vi "Step.vi"(8 "error in (no error)":errorcluster, 11 "SQL Statement in":refnum<class "SQL Statement.lvclass">) -> (0 "error out":errorcluster, 2 "Row returned":bool, 3 "SQL Statement out":refnum<class "SQL Statement.lvclass">)   [LabVIEW 2023, in "SQLiteSupport.lvlib" / "SQL Statement.lvclass"]
doc: "Steps to another row of a multiple-row returned data set. Please use \"First Step\" to actually execute the statement (and return the first row), rather than \"Step\"."
uses:
  SQL Statement.lvclass
panel:
  # "Step, and anything containing Step, may block while\nwaiting for another operation to unlock the database,\nand thus must be reentrant in order to prevent lock-up."
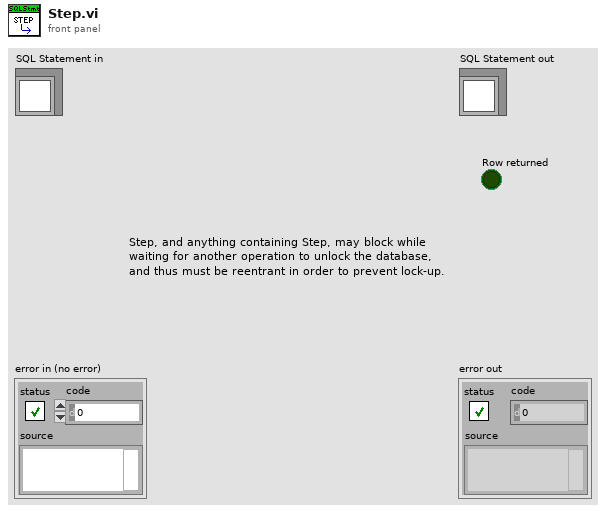
[diagram p1: front panel]
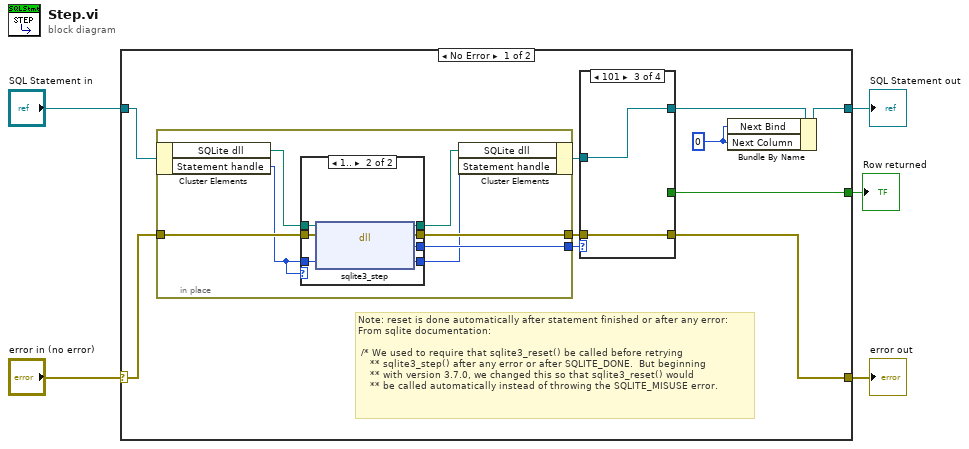
[diagram p0: block diagram]
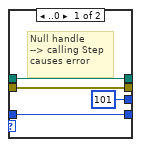
[diagram p2: hidden frame]
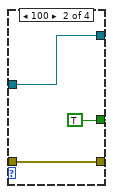
[diagram p4: hidden frame]
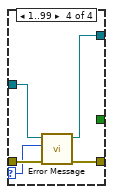
[diagram p5: hidden frame]
diagram:
  n1 = case shown="No Error" "error in (no error)" {
    selector: "error in (no error)" -> [w15 w47]
    tunnel: [w13 w47] -> w4
    tunnel: [w10 w46] -> w2
    tunnel: "SQL Statement in" -> [w7 w46]
    tunnel: [w11 _] -> w1
    frame No Error {
      w9 = 0 ("Next Column")
      # "Note: reset is done automatically after statement finished or after any error:\nFrom sqlite documentation:\n\n /* We used to require that sqlite3_reset() be called before retrying\n    ** sqlite3_step() after any error or after SQLITE_DONE.  But beginning\n    ** with version 3.7.0, we changed this so that sqlite3_reset() would\n    ** be called automatically instead of throwing the SQLITE_MISUSE error."
      n2 = in-place {
        in-place-border: w15 -> [w22]
        in-place-border: [w21] -> w14
        in-place-border: [w20] -> w12
        n3 = in-place-cluster #1(w7) -> ("SQLite dll"=w19:path, "Statement handle"=w16:u64)
        n4 = case shown="1.." w16 {
          tunnel: w22 -> [w25 w33]
          tunnel: [w25 w32] -> w21
          tunnel: [101 ("return code") w31] -> w20
          tunnel: w19 -> [w26 w30]
          tunnel: w16 -> [w23 w29]
          tunnel: [w23 w28] -> w18
          tunnel: [w26 w27] -> w17
          frame ..0 {
            # "Null handle\n--> calling Step\ncauses error"
          }
          frame 1.. {
            n5 = dll-call lib="C:/SQLite/sqlite3.dll" fn="sqlite3_step"(path in=w30, error in=w33, "Statement"=w29) -> (path out=w27:path, error out=w32:errorcluster, "return code"=w31:i32, "Statement"=w28:u64)  [unwired: 1 in]
          }
        }
        n6 = in-place-cluster #1("SQLite dll"=w17, "Statement handle"=w18) -> (w6:refnum<class "SQL Statement.lvclass">)
      }
      n7 = case shown="101" w12 {
        selector: w12 -> [_ _ _ w41]
        tunnel: w14 -> [w35 w37 w40 w45]
        tunnel: [w35 w37 w40 w44] -> w13
        tunnel: [_ TRUE _ _] -> w11
        tunnel: w6 -> [w34 w36 w39 w43]
        tunnel: [w34 w36 w39 w42] -> w8
        frame 0, Default {
        }
        frame 100 {
        }
        frame 101 {
        }
        frame 1..99 {
          n8 = call "Error Message.vi"("error in (no error)"=w45, "error code"=w41, "SQL Statement In"=w43) -> ("error out"=w44:errorcluster, "SQL Statement Out"=w42:refnum<class "SQL Statement.lvclass">)  [unwired: 7 in]
        }
      }
      n9 = Bundle By Name(cluster=w8, "Next Bind"=w9, "Next Column"=w9) -> (w10:refnum<class "SQL Statement.lvclass">)
    }
    frame Error {
    }
  }
  "error out" <- w4
  "SQL Statement out" <- w2
  "Row returned" <- w1
